vi "Initialize.vi"(8 "error in (no error)":errorcluster, 11 "Shifter-ShiftHigh-Cmd in":refnum<class "SF-ShiftHigh-Cmd.lvclass">) -> (0 "error out":errorcluster, 3 "Shifter-ShiftHigh-Cmd out":refnum<class "SF-ShiftHigh-Cmd.lvclass">)   [LabVIEW 2013, in "SF-ShiftHigh-Cmd.lvclass"]
uses:
  SF-ShiftHigh-Cmd.lvclass
  States/SF-HighSpeed-State/Shifter-HighSpeed.lvclass
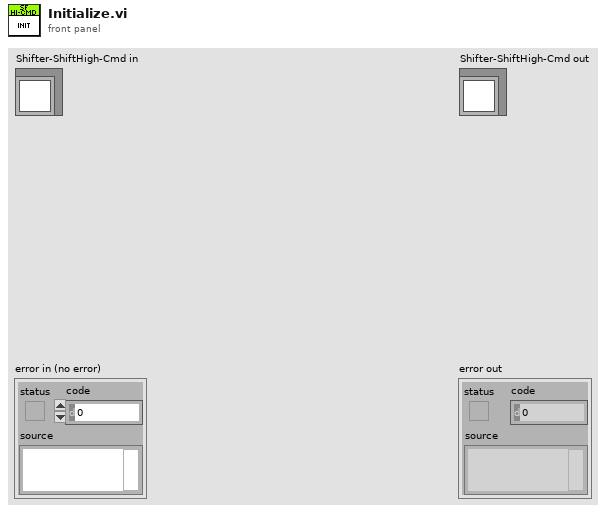
[diagram p1: front panel]
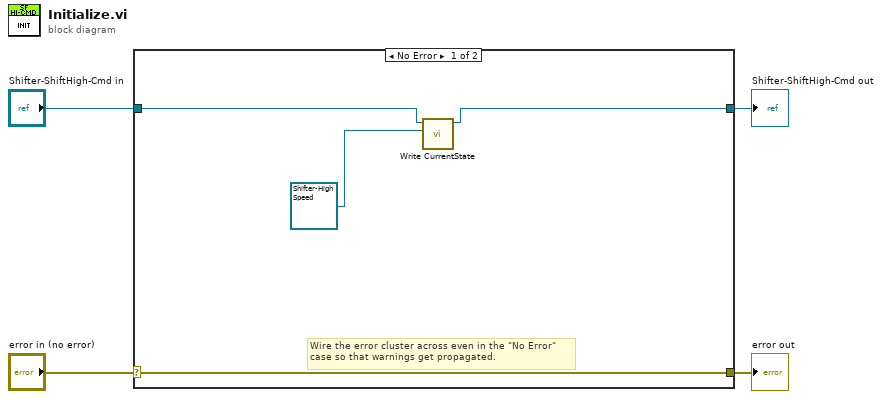
[diagram p0: block diagram]
diagram:
  n1 = case shown="No Error" "error in (no error)" {
    selector: "error in (no error)" -> [w8 w10]
    tunnel: [w8 w10] -> w3
    tunnel: [w6 w9] -> w1
    tunnel: "Shifter-ShiftHigh-Cmd in" -> [w7 w9]
    frame No Error {
      # "Wire the error cluster across even in the \"No Error\"\ncase so that warnings get propagated."
      n2 = call-dynamic "Write CurrentState.vi"("State.lvclass"=refnum<class "Shifter-HighSpeed.lvclass"> refnum ("Shifter-HighSpeed.lvclass"), "Command in"=w7) -> ("Command out"=w6:refnum<class "SF-ShiftHigh-Cmd.lvclass">)  [unwired: 8 in, 1 out]
    }
    frame Error {
    }
  }
  "error out" <- w3
  "Shifter-ShiftHigh-Cmd out" <- w1
